vi "Essai mesure time.vi"() -> ()   [LabVIEW 2020]
panel:
  out "Delta T":u32 format="%.0f ms"
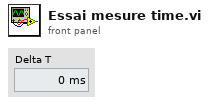
[diagram p1: front panel]
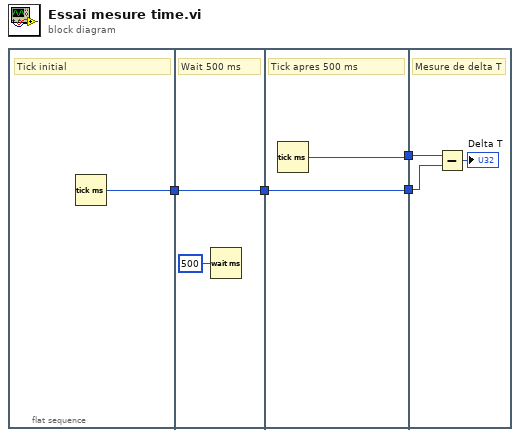
[diagram p0: block diagram]
diagram:
  n1 = flat-sequence {
    tunnel: [w5] -> w4
    tunnel: w4 -> [w6]
    tunnel: [w6] -> w3
    tunnel: w3 -> [w9]
    tunnel: [w9] -> w2
    tunnel: [w8] -> w1
    tunnel: w2 -> [w11]
    tunnel: w1 -> [w12]
    frame #0 {
      # "Tick initial"
      n2 = Tick Count (ms)() -> (millisecond timer value=w5:u32)
    }
    frame #1 {
      # "Wait 500 ms"
      n3 = Wait (ms)(milliseconds to wait=u32 500 ("attente (ms)")) -> ()  [unwired: 1 out]
    }
    frame #2 {
      # "Tick apres 500 ms"
      n4 = Tick Count (ms)() -> (millisecond timer value=w8:u32)
    }
    frame #3 {
      # "Mesure de delta T"
      n5 = Subtract(x=w12, y=w11) -> (x-y=→"Delta T":u32)
    }
  }
